vi "Buffered Log Sink Example.vi"() -> ()   [LabVIEW 2019, in "Logger Examples.lvlib"]
uses:
  Logger Examples.lvlib
  Source/Composed Log/Types/Log Level.ctl
  Source/String Formats/String Expression Format/String Expression Format.lvclass/String Expression Format.ctl
  Source/Composed Log/LoggerReference/LoggerReference.lvclass/LoggerReference.ctl
  601d143e-8928-4a3b-9174-3083e729aaa9.vi
  Source/String Formats/String Expression Format/Run Formatter.vi
  Source/Composed Log/LoggerReference/Return Aggregate Queues.vi
  Source/Composed Log/LoggerReference/Add Aggregate Log.vi
  601d143e-8928-4a3b-9174-3083e729aaa9.vi/16370e4d-f3cd-41c1-a9a1-4fb3403731d5.vi
  Source/Composed Log/LoggerReference/Log.vi
  Source/Composed Log/LoggerReference/Get Valid Event Time.vi
  <vilib>/dlg_ctls.llb/Space Constant.vi
  Source/Composed Log/LoggerReference/Send Add Sink.vi
  Source/Composed Log/LoggerReference/Remove Stale Logs.vi
  Source/String Formats/String Expression Format/String Expression Format.lvclass
  C:/CS/Log/Source/IStringFormat/IStringFormat.lvclass
  Source/String Control Sink/String Control Sink.lvclass
  C:/CS/Log/Source/Composed Log/Log Sink/Log Sink.lvclass
  Source/Buffered Log Sink/Buffered Log Sink.lvclass
  Source/Composed Log/Application Logger/Launch Worker Loop.vi
  Source/Composed Log/LoggerReference/Initialize Logger Instance.vi
  Source/Composed Log/LoggerReference/LoggerReference.lvclass
  Source/Composed Log/IErrorFormat/IErrorFormat.lvclass
  Source/Composed Log/Log Sink/Log Sink.lvclass
  Source/Composed Log/Composed Log.lvlib
  C:/CS/Log/Source/String Log Sink/String Log Sink.lvclass
  Source/Buffered String Log Sink/Buffered String Log Sink.lvclass
panel:
  in  "Log Error":bool
  in  "Error Information":string
  in  "Error Code":i32
  in  "Event Level":T1(ring)
  out "1S Timeout, 5 Element Buffer":string
  out "No Timeout - 5 Element Buffer":string
  out "500mS Timeout, Unlimited Buffer":string
  in  "Data To Log":string
  in  "Source":string="User"
  in  "Log":bool
  # "This Sink will only log events once its buffer is full. Any unlogged events will be logged on shutdown."
  # "This Sink will only log events once its timer elapses. Any unlogged events will be logged on shutdown."
  # "This Sink will log events when its buffer is full, or its timer elapses. Any unlogged events will be logged on shutdown."
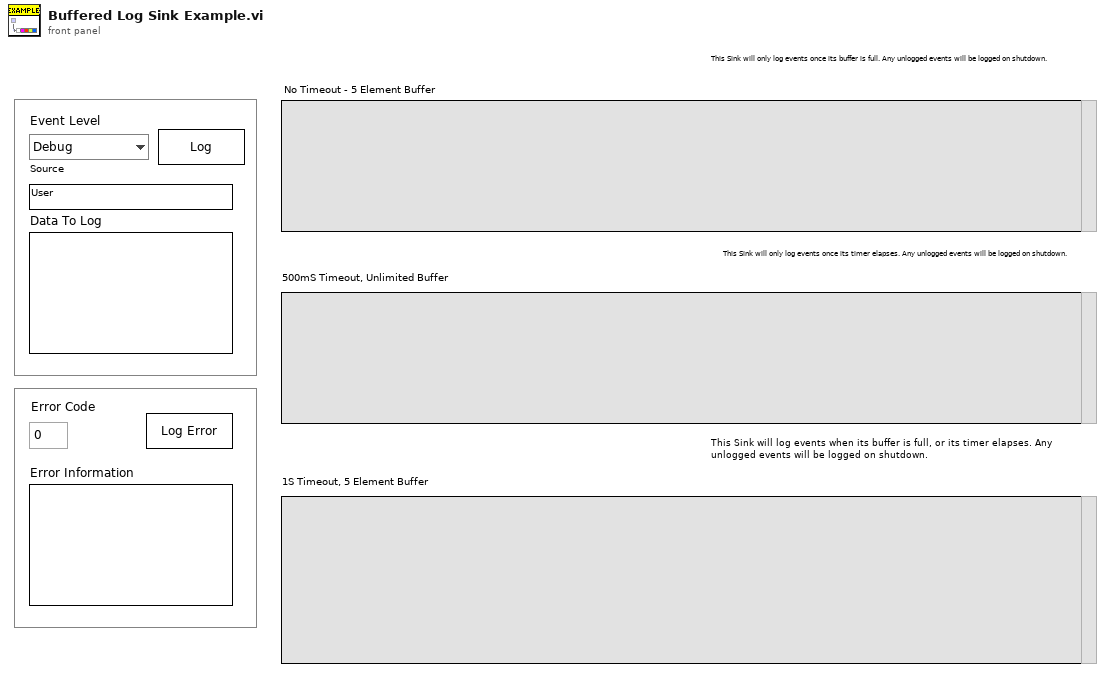
[diagram p1: front panel]
types:
  T1 = enum16{"Debug", "Info", "Warning", "Error", "Critical"}
  T2 = typedef "Composed Log.lvlib/Log Level.ctl" = enum16{"Debug", "Info", "Warning", "Error", "Critical"}
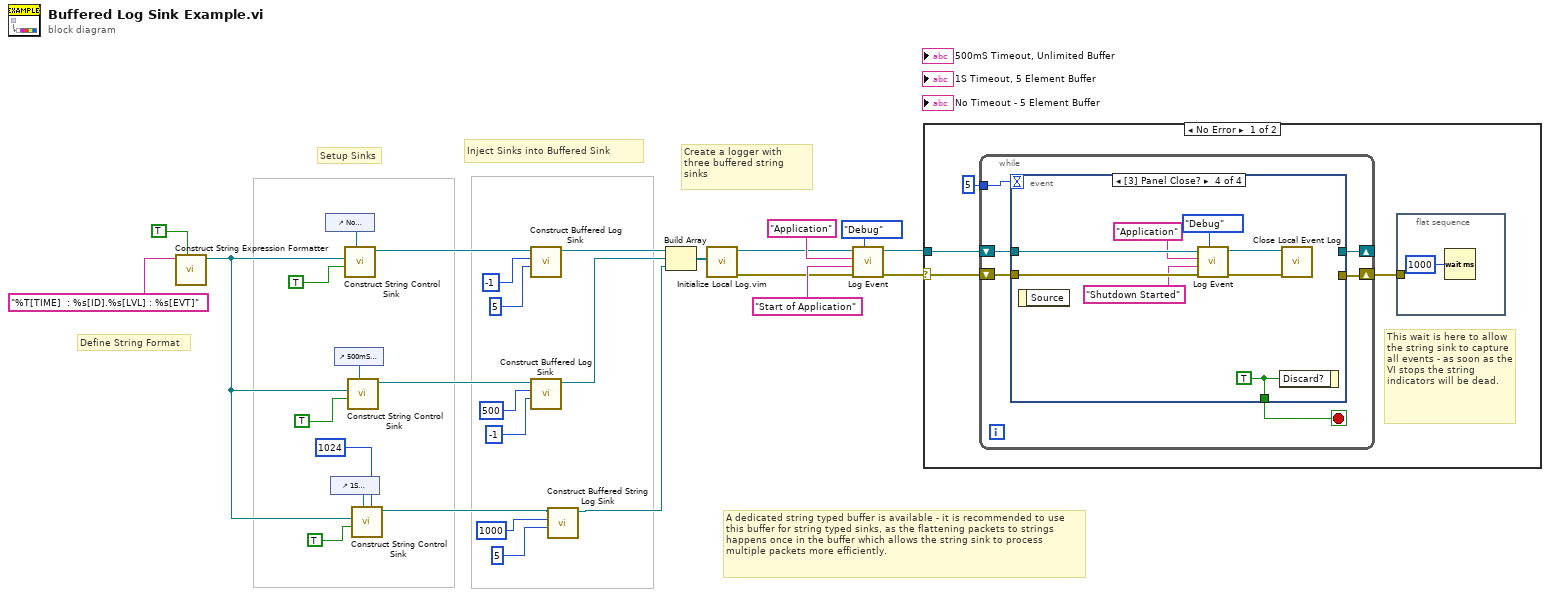
[diagram p0: block diagram]
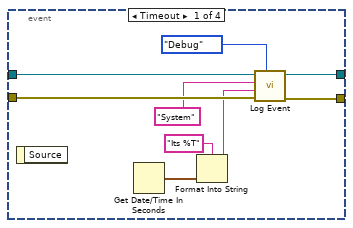
[diagram p2: hidden frame]
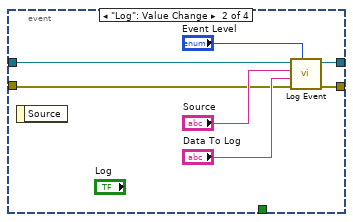
[diagram p3: hidden frame]
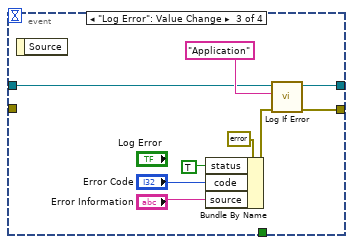
[diagram p4: hidden frame]
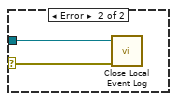
[diagram p5: hidden frame]
diagram:
  # "A dedicated string typed buffer is available - it is recommended to use this buffer for string typed sinks, as the flattening packets to strings happens once in the buffer which allows the string sink to process multiple packets more efficiently."
  # "Inject Sinks into Buffered Sink"
  # "Setup Sinks"
  # "Define String Format"
  # "Create a logger with three buffered string sinks"
  n1 = call "Construct String Expression Formatter.vi"("Append EOL?"=TRUE, "Format Specifier"="%T[TIME]  : %s[ID].%s[LVL] : %s[EVT]") -> ("String Expression Format out"=w6:refnum<class "String Expression Format.lvclass">)  [unwired: 8 in, 1 out]
  n2 = control-ref of="No Timeout - 5 Element Buffer"() -> (w28:refnum<vi>)
  n3 = control-ref of="1S Timeout, 5 Element Buffer"() -> (w25:refnum<vi>)
  n4 = control-ref of="500mS Timeout, Unlimited Buffer"() -> (w29:refnum<vi>)
  n5 = call "Construct String Control Sink.vi"("Str Refnum"=w28, "AutoScroll?(F)"=TRUE, "LogFormat"=w6) -> ("String Control Sink out"=w14:refnum<class "String Control Sink.lvclass">)  [unwired: 8 in]
  n6 = call "Construct String Control Sink.vi"("Str Refnum"=w29, "AutoScroll?(F)"=TRUE, "LogFormat"=w6) -> ("String Control Sink out"=w10:refnum<class "String Control Sink.lvclass">)  [unwired: 8 in]
  n7 = call "Construct String Control Sink.vi"("Buffer Length(0)"=1024, "Str Refnum"=w25, "AutoScroll?(F)"=TRUE, "LogFormat"=w6) -> ("String Control Sink out"=w3:refnum<class "String Control Sink.lvclass">)  [unwired: 7 in]
  n8 = call "Construct Buffered Log Sink.vi"("Buffer Size (128)"=5, "Buffer Timeout ms (-1)"=-1, "Sink to Buffer"=w14) -> ("Buffered Log Sink out"=w13:refnum<class "Buffered Log Sink.lvclass">)  [unwired: 8 in]
  n9 = call "Construct Buffered Log Sink.vi"("Buffer Size (128)"=-1, "Buffer Timeout ms (-1)"=500, "Sink to Buffer"=w10) -> ("Buffered Log Sink out"=w9:refnum<class "Buffered Log Sink.lvclass">)  [unwired: 8 in]
  n10 = call "Construct Buffered String Log Sink.vi"("Buffer Size (128)"=5, "Buffer Timeout ms (-1)"=1000, "Sink Type"=w3) -> ("Buffered String Log Sink out"=w4:refnum<class "Buffered String Log Sink.lvclass">)  [unwired: 8 in]
  n11 = Build Array(w13, w9, w4) -> (w15:refnum<class "Log Sink.lvclass">[])
  n12 = call "Initialize Local Log.vim"("Startup Sink(s)"=w15) -> ("error out"=w21:errorcluster, "Log Instance Reference"=w20:refnum<class "LoggerReference.lvclass">)  [unwired: 8 in, 1 out]
  n13 = call "Log Event.vi"("Event Level"=Log_Level."Debug", "error in (no error)"=w21, "Data To Log"="Start of Application", "SourceID"="Application", "Log Instance"=w20) -> ("error out"=w19:errorcluster, "Log Instance Out"=w18:refnum<class "LoggerReference.lvclass">)  [unwired: 5 in]
  n14 = case shown="No Error" w19 {
    selector: w19 -> [w33 w75]
    tunnel: w18 -> [w34 w76]
    frame No Error {
      # "This wait is here to allow the string sink to capture all events - as soon as the VI stops the string indicators will be dead."
      n15 = while {
        shift-right: [w39] -> _
        shift-left: w34 -> [w40]
        shift-right: [w37] -> w31
        shift-left: w33 -> [w38]
        tunnel: 5 -> [w36]
        stop <- w41 stop-if-true
        n16 = event shown="[3] Panel Close?" {
          selector: _ -> [_ _ _ _]
          dyn-events: _ -> [_ _ _ _]
          timeout: w36 -> [_ _ _ _]
          tunnel: [_ _ _ w74] -> w41
          tunnel: w40 -> [w50 w54 w60 w72]
          tunnel: [w49 w52 w58 _] -> w39
          tunnel: w38 -> [w47 w51 _ w73]
          tunnel: [w46 w53 w59 _] -> w37
          event Timeout {
            n17 = event-data() -> ()  [unwired: 1 in, 1 out]
            n18 = Get Date/Time In Seconds() -> (seconds since 1Jan1904=w44:timestamp)
            n19 = Format Into String(format string="Its %T" ("Log Message"), w44) -> (resulting string=w42:string)  [unwired: 2 in, 1 out]
            n20 = call "Log Event.vi"("Event Level"=Log_Level."Debug", "error in (no error)"=w47, "Data To Log"=w42, "SourceID"="System" ("Event Source"), "Log Instance"=w50) -> ("error out"=w46:errorcluster, "Log Instance Out"=w49:refnum<class "LoggerReference.lvclass">)  [unwired: 5 in]
          }
          event "Log": Value Change {
            n21 = event-data() -> ()  [unwired: 1 in, 1 out]
            n22 = call "Log Event.vi"("Event Level"="Event Level", "error in (no error)"=w51, "Data To Log"="Data To Log", "SourceID"="Source", "Log Instance"=w54) -> ("error out"=w53:errorcluster, "Log Instance Out"=w52:refnum<class "LoggerReference.lvclass">)  [unwired: 5 in]
          }
          event "Log Error": Value Change {
            n23 = event-data() -> ()  [unwired: 1 in, 1 out]
            n24 = Bundle By Name(cluster=errorcluster {"status"=FALSE, "code"=0, "source"=""} ("Error In"), "status"=TRUE, "code"="Error Code", "source"="Error Information") -> (w64:errorcluster)
            n25 = call "Log If Error.vi"("Error In"=w64, "SourceID"="Application" ("Source"), "Log Instance"=w60) -> ("error out"=w59:errorcluster, "Log Instance Out"=w58:refnum<class "LoggerReference.lvclass">)  [unwired: 7 in]
          }
          event Panel Close? {
            w74 = TRUE ("Discard?")
            n26 = event-data() -> ()  [unwired: 1 in, 1 out]
            n27 = call "Log Event.vi"("Event Level"=Log_Level."Debug", "error in (no error)"=w73, "Data To Log"="Shutdown Started", "SourceID"="Application", "Log Instance"=w72) -> ("error out"=w71:errorcluster, "Log Instance Out"=w70:refnum<class "LoggerReference.lvclass">)  [unwired: 5 in]
            n28 = event-data("Discard?"=w74) -> ()  [unwired: 1 in, 1 out]
            n29 = call "Close Local Event Log.vi"("error in (no error)"=w71, "Log Instance"=w70) -> ()  [unwired: 9 in, 1 out]
          }
        }
      }
      n30 = flat-sequence {
        tunnel: w31 -> [_]
        frame #0 {
          n31 = Wait (ms)(milliseconds to wait=u32 1000) -> ()  [unwired: 1 out]
        }
      }
    }
    frame Error {
      n32 = call "Close Local Event Log.vi"("error in (no error)"=w75, "Log Instance"=w76) -> ()  [unwired: 9 in, 1 out]
    }
  }
